vi "Set SG Path.vi"(0 "Path in":refnum<class "SA Path.lvclass">, 5 "Cal point in":T1, 11 "error in":errorcluster) -> (4 "Path out":refnum<class "SA Path.lvclass">, 6 "Cal point out":T1, 8 "Source Gain":dbl, 10 "Digital Gain":dbl, 15 "error out":errorcluster)   [LabVIEW 2023, in "RFFixtureCharact.RMM.lvlib" / "SA Path.lvclass"]
uses:
  SA Path.lvclass
  Public/Base Classes/Scalar/Scalar Path/Type Definitions/Cal Point.ctl
  <vilib>/addons/_RFCalAndCharactDatabase/NI_RFCalAndCharact_Database_API.lvlibp/Characterization/Controls/Type.ctl
  Public/Base Classes/Scalar/SA Abstract Path/SA Abstract Path.lvclass/SA Abstract Path.ctl
  Public/Base Classes/Scalar/SA Abstract Path/Properties/Read Cal Tone Pin.vi
  Public/Base Classes/Scalar/SA Path/SA Path.lvclass
  SA Path.lvclass/SA Path.ctl
  <instrlib>/niRFSG/niRFSG.llb/niRFSG Create De-embedding S-parameter Table (array).vi
  <vilib>/addons/_RFCalAndCharactDatabase/NI_RFCalAndCharact_Database_API.lvlibp/Characterization/Characterization.lvlib
  Public/Base Classes/Scalar/Scalar Path/Scalar Path.lvclass
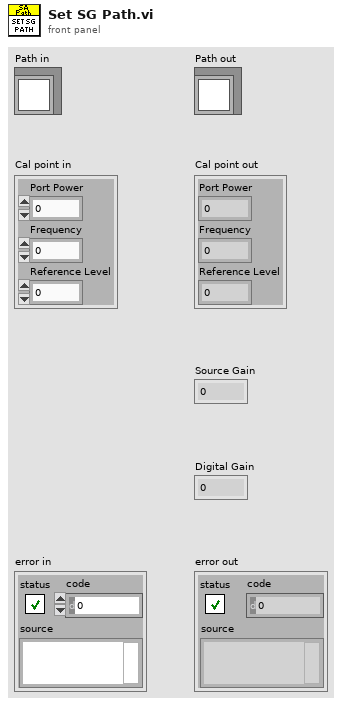
[diagram p1: front panel]
types:
  T1 = typedef "RFFixtureCharact.Public.lvlib/Scalar Path.lvclass/Cal Point.ctl" = cluster{"Port Power":dbl, "Frequency":dbl, "Reference Level":dbl}
  T2 = typedef "NI_RFCalAndCharact_Database_API.lvlibp/Characterization.lvlib/Type.ctl" = u16
  T3 = typedef "NI_RFCalAndCharact_Database_API.lvlibp/Characterization.lvlib/Path Handle.ctl" = refnum<k24>
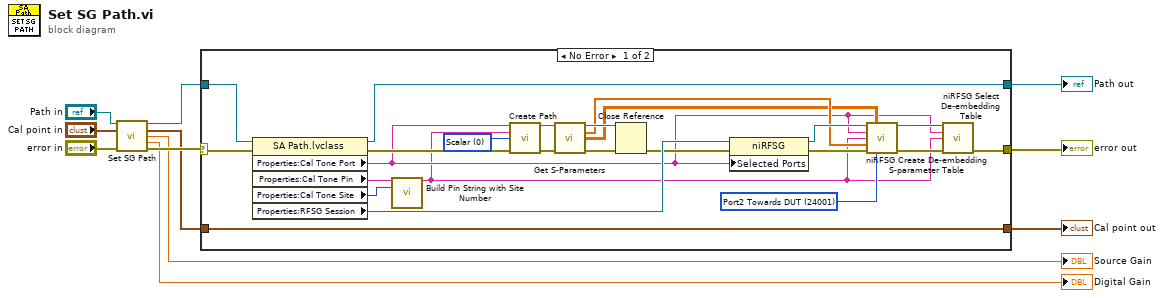
[diagram p0: block diagram]
diagram:
  n1 = call-parent "Set SG Path.vi"("Path in"="Path in", "Cal point in"="Cal point in", "error in (no error)"="error in") -> ("Path out"=w10:refnum<class "SA Path.lvclass">, "Cal point out"=w9:T1, "Source Gain"=→"Source Gain":dbl, "Digital Gain"=→"Digital Gain":dbl, "error out"=w11:errorcluster)  [unwired: 8 in]
  n2 = case shown="No Error" w11 {
    selector: w11 -> [w13 w38]
    tunnel: w10 -> [w16 w37]
    tunnel: [w15 w37] -> w5
    tunnel: [w14 w38] -> w4
    tunnel: [w12 w36] -> w3
    tunnel: w9 -> [w12 w36]
    frame No Error {
      w21 = 24001 items=["Port1 Towards DUT"=24000, "Port2 Towards DUT"=24001] ("S-parameters orientation")
      w34 = T2 0 items=["Scalar", "Vector"] ("Type")
      n3 = property class="SA Path.lvclass"(reference=w16, error in=w13) -> (reference out=w15:refnum<class "SA Path.lvclass">, error out=w31:errorcluster, "Properties:Cal Tone Port"=w18:string, "Properties:Cal Tone Pin"=w30:string, "Properties:Cal Tone Site"=w29:i32, "Properties:RFSG Session"=w35:refnum<k15>)
      n4 = call <vilib>:"Build Pin String with Site Number.vi"("Pin Name"=w30, "Site Number"=w29) -> ("Pin String"=w17:string)  [unwired: 13 in]
      n5 = call <vilib>:"Create Path.vi"("Port 1"=w18, "Port 2"=w17, "Type"=w34, "error in"=w31) -> ("Path"=w33:T3, "error out"=w32:errorcluster)  [unwired: 10 in]
      n6 = call <vilib>:"Get S-Parameters.vi"("Path In"=w33, "error in"=w32) -> ("Path Out"=w25:T3, "Frequencies (Hz)"=w23:dbl[], "S-Parameters"=w22:cdb[][][], "error out"=w26:errorcluster)  [unwired: 10 in]
      n7 = Close Reference(reference=w25, error in (no error)=w26) -> (error out=w24:errorcluster)
      n8 = property class="niRFSG"(reference=w35, error in=w24, "Selected Ports"=w18) -> (reference out=w27:refnum<k15>, error out=w28:errorcluster)
      n9 = call-poly <instrlib>:"niRFSG Create De-embedding S-parameter Table.vi"("instrument handle"=w27, "S-parameter table"=w22, "port"=w18, "table name"=w17, "frequencies"=w23, "error in"=w28, "S-parameters orientation"=w21) -> ("instrument handle out"=w19:refnum<k15>, "error out"=w20:errorcluster)  [unwired: 7 in]
      n10 = call <instrlib>:"niRFSG Select De-embedding Table.vi"("instrument handle"=w19, "port"=w18, "table name"=w17, "error in"=w20) -> ("error out"=w14:errorcluster)  [unwired: 10 in, 1 out]
    }
    frame Error {
    }
  }
  "error out" <- w4
  "Cal point out" <- w3
  "Path out" <- w5
